vi "EncoderStartStop_Simulation_Global.vi"(0 "menu":enum16{"set", "get", "delete"}(ring)=enum."get", 5 "Encoder Index":T1, 7 "start/stop in":bool, 11 "error in (no error)":errorcluster) -> (8 "start/stop out":bool, 15 "error out":errorcluster)   [LabVIEW 2017]
doc: "Sets a reference into a registry, gets a reference from a registry, or deletes a reference from a registry. The reference is accessed by name, and can be given any unique name.\n\nThis software is licensed. Open the labview\\readme\\WPI Robotics Library Open Source License.txt file for more information."
uses:
  <vilib>/Rock Robotics/SystemInterfaces/Encoder/FPGA_EncoderIdx.ctl
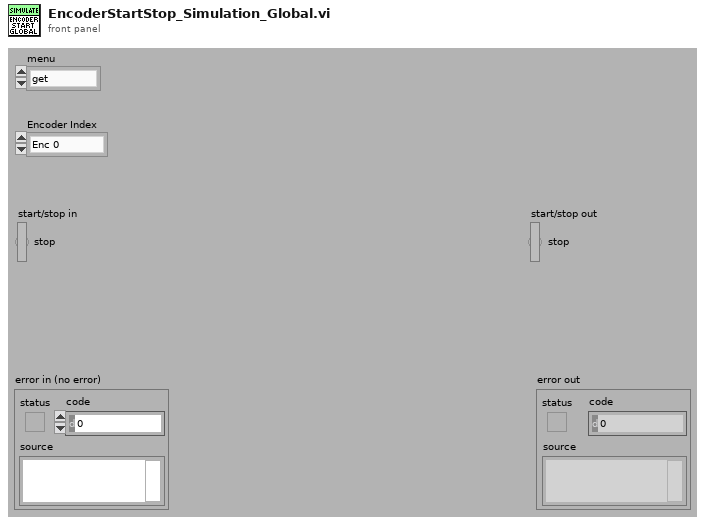
[diagram p1: front panel]
types:
  T1 = typedef "FPGA_EncoderIdx.ctl" = enum8{"Enc 0", "Enc 1", "Enc 2", "Enc 3", "Enc 4", "Enc 5", "Enc 6", "Enc 7", "Invalid"}
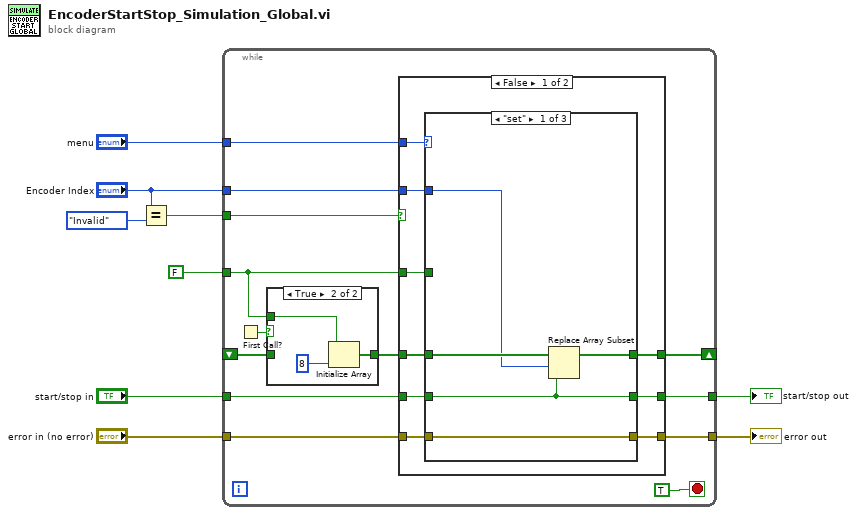
[diagram p0: block diagram]
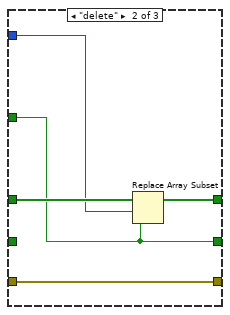
[diagram p2: hidden frame]
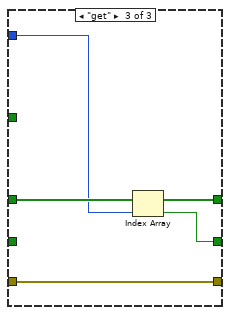
[diagram p3: hidden frame]
diagram:
  n1 = Equal?(x="Encoder Index", y=FPGA_EncoderIdx."Invalid" ("Encoder")) -> (x = y?=w4:bool)
  n2 = while {
    tunnel: "start/stop in" -> [w22]
    tunnel: "error in (no error)" -> [w18]
    shift-right: [w21] -> _
    shift-left: _ -> [w13]
    tunnel: [w20] -> w1
    tunnel: "menu" -> [w19]
    tunnel: [w17] -> w8
    tunnel: "Encoder Index" -> [w12]
    tunnel: w4 -> [w11]
    tunnel: FALSE -> [w10]
    stop <- TRUE stop-if-true
    n3 = First Call?() -> (First Call?: T/F=w15:bool)
    n4 = case shown="True" w15 {
      tunnel: [w49 w51] -> w14
      tunnel: w13 -> [w49 _]
      tunnel: w10 -> [_ w50]
      frame False {
      }
      frame True {
        n5 = Initialize Array(w50, 8 ("dimension size")) -> (w51:bool[])
      }
    }
    n6 = case shown="False" w11 {
      tunnel: w22 -> [w31 _]
      tunnel: [w30 w48] -> w21
      tunnel: [w29 w46] -> w20
      tunnel: w19 -> [w28 _]
      tunnel: w18 -> [w27 w47]
      tunnel: [w26 w47] -> w17
      tunnel: w14 -> [w25 w48]
      tunnel: w12 -> [w24 _]
      tunnel: w10 -> [w23 w46]
      frame False {
        n7 = case shown="\"set\"" w28 {
          tunnel: w31 -> [w34 _ _]
          tunnel: [w35 w40 w45] -> w30
          tunnel: w25 -> [w36 w41 w45]
          tunnel: [w34 w38 w44] -> w29
          tunnel: [w33 w39 w43] -> w26
          tunnel: w27 -> [w33 w39 w43]
          tunnel: w24 -> [w32 w37 w42]
          tunnel: w23 -> [_ w38 _]
          frame "set" {
            n8 = Replace Array Subset(array=w36, new element=w34, index=w32) -> (w35:bool[])
          }
          frame "delete" {
            n9 = Replace Array Subset(array=w41, new element=w38, index=w37) -> (w40:bool[])
          }
          frame "get" {
            n10 = Index Array(array=w45, index=w42) -> (element=w44:bool)
          }
        }
      }
      frame True {
        # "Do nothing if channel is Invalid."
      }
    }
  }
  "error out" <- w8
  "start/stop out" <- w1
